vi "AddNewTSMProperty.vi"(9 "Target Class":path=path "GlobalTestData.lvclass", 10 "Property Scope":enum16{"Global", "PerSite"}(ring), 11 "Property Name":string) -> (0 "error out":errorcluster)   [LabVIEW 2019]
doc: "This VI will add a new Global (default) or Per-Site TSM-based property to the target class (default: GlobalTestData.lvclass). \nThis VI must be placed relative to the target class (same directory, or at a higher level).\nThis VI should not be added to, or claimed by, the target class (this is not the intended use case, you will get a lock-out error)."
uses:
  <vilib>/regexp/Match Regular Expression.xnode
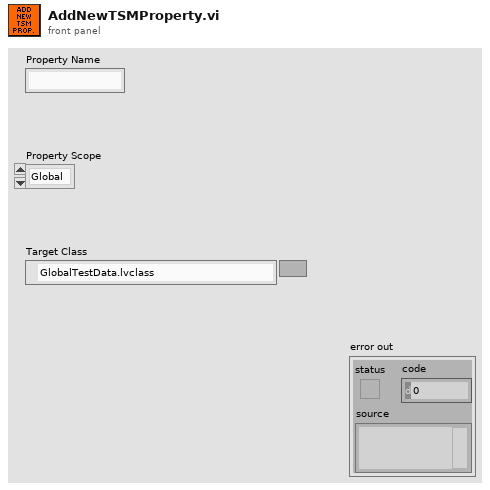
[diagram p1: front panel]
types:
  T1 = typedef "LIBUIP_item_type.ctl" = enum16{"None", "ParentLib", "Property Def Item", "VI", "Non-VI", "Folder", "Library", "Menu", "XI Ability VI", "XI Method VI", "XI Property VI", "Property Folder", "Class Private Data"}
  T2 = enum16{"Invalid Wire Rule", "Required", "Recommended", "Optional", "Dynamic Dispatch"}[]
  T3 = enum16{"Invalid Wire Rule", "Required", "Recommended", "Optional", "Dynamic Dispatch"}
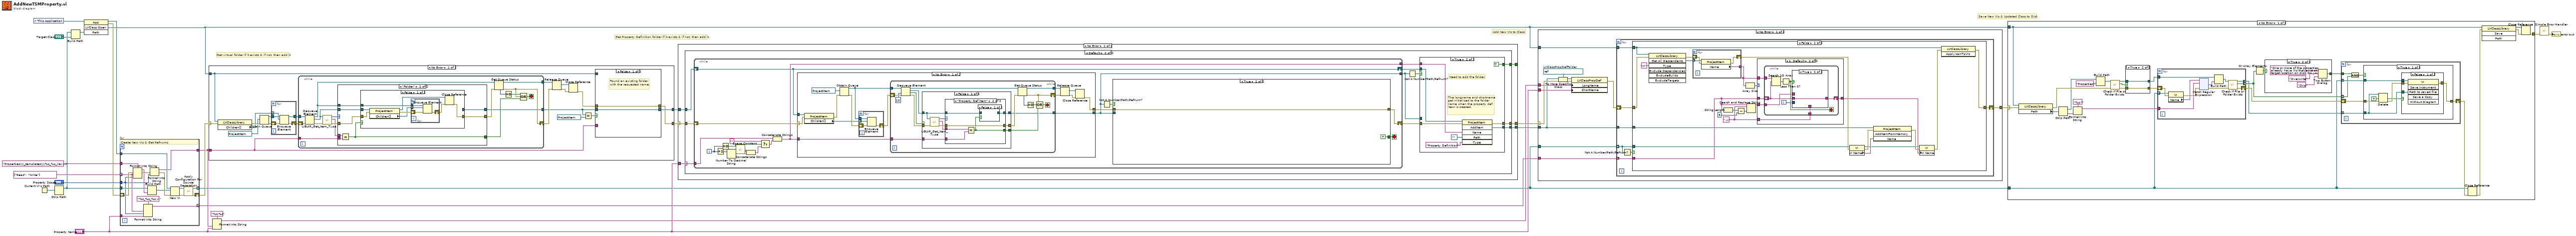
[diagram p0: block diagram]
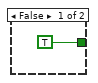
[diagram p2: hidden frame]
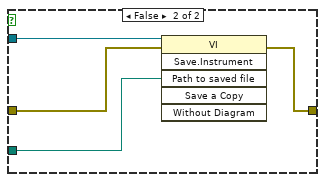
[diagram p4: hidden frame]
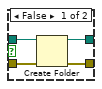
[diagram p5: hidden frame]
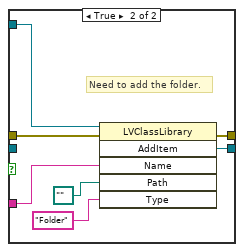
[diagram p7: hidden frame]
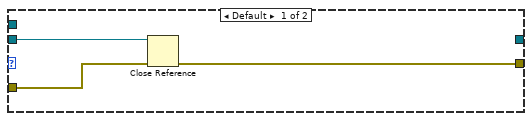
[diagram p8: hidden frame]
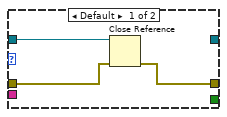
[diagram p12: hidden frame]
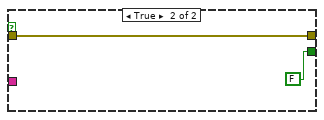
[diagram p14: hidden frame]
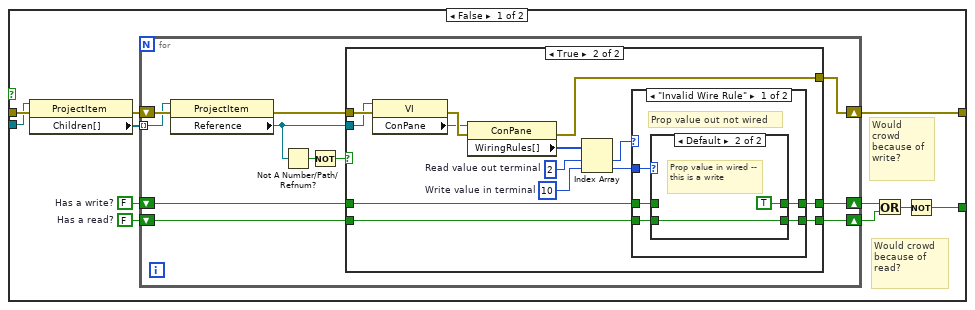
[diagram p16: hidden frame]
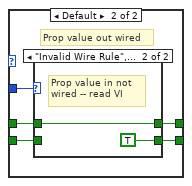
[diagram p19: hidden frame]
diagram:
  # "Add New VIs to Class"
  # "Save New VIs & Updated Class to Disk"
  # "Get Property Definition folder if it exists & if not, then add it"
  # "Get virtual folder if it exists & if not, then add it"
  n1 = control-ref of="This Application"() -> (w25:refnum<vi>)
  n2 = Current VI's Path() -> (path=w24:path)
  n3 = Strip Path(path=w24) -> (stripped path=w1:path)  [unwired: 1 out]
  n4 = Build Path(base path=w1, name or relative path="Target Class") -> (appended path=w3:path)
  n5 = invoke on="Invoke Node" class="App" method="LVClass.Open"(reference=w25, "Path"=w3) -> (reference out=w13:refnum<vi>, error out=w10:errorcluster, "LVClass.Open"=w16:refnum<vi>)  [unwired: 2 in, 1 out]
  n6 = for {
    tunnel: w1 -> [w42]
    tunnel: "Properties\\\\_templates\\\\%s_%s_Var.vit" -> [w41]
    tunnel: string[] ["Read", "Write"] -> [w31] mode=indexing
    tunnel: "Property Scope" -> [w30]
    tunnel: "Property Name" -> [w29]
    tunnel: w13 -> [w40]
    tunnel: [w39] -> w4 mode=indexing
    tunnel: [w35] -> w8
    shift-right: [w34] -> w15
    shift-left: w10 -> [w43]
    tunnel: [w27] -> w5 mode=indexing
    # "Create New VIs & Get Refnums"
    n7 = Format Into String(format string=w41, error in=w43, w31, w30) -> (resulting string=w28:string, error out=w38:errorcluster)  [unwired: 1 in]
    n8 = Format Into String(format string="%s_%s_%s.vi", w31, w30, w29) -> (resulting string=w27:string)  [unwired: 2 in, 1 out]
    n9 = Build Path(base path=w42, name or relative path=w28) -> (appended path=w33:path)
    n10 = Format Into String(error in=w38, w30) -> (resulting string=w35:string, error out=w37:errorcluster)  [unwired: 2 in]
    n11 = New VI(8:w37, 10:w33, 11:w40) -> (0:w26:errorcluster, 3:w36:refnum<vi>)  [unwired: 4 in]
    n12 = call <vilib>:"Apply Configuration For Source Separation.vi"("error in (no error)"=w26, "VI in"=w36) -> ("error out"=w34:errorcluster, "VI out"=w39:refnum<vi>)  [unwired: 8 in]
  }
  n13 = case shown="No Error" w15 {
    selector: w15 -> [w54 w120]
    tunnel: w8 -> [w45 _]
    tunnel: w16 -> [w44 _]
    tunnel: [w47 _] -> w23
    tunnel: [w46 w120] -> w22
    frame No Error {
      n14 = property class="LVClassLibrary"(reference=w44, error in=w54) -> (error out=w59:errorcluster, "Children[]"=w53:refnum<vi>[])  [unwired: 1 out]
      n15 = Obtain Queue(element data type=refnum<vi> refnum ("ProjectItem Refnum"), error in (no error)=w59) -> (queue out=w63:refnum<queue>, error out=w62:errorcluster)  [unwired: 2 in, 2 out]
      n16 = for {
        tunnel: w53 -> [w76] mode=indexing
        tunnel: w63 -> [w77]
        tunnel: [w73] -> w61
        shift-right: [w74] -> w60
        shift-left: w62 -> [w75]
        n17 = Enqueue Element(queue=w77, element=w76, error in (no error)=w75) -> (queue out=w73:refnum<queue>, error out=w74:errorcluster)  [unwired: 2 out]
      }
      n18 = while {
        tunnel: w61 -> [w92]
        shift-right: [w78] -> w55
        shift-left: w60 -> [w93]
        tunnel: [w79] -> w58
        tunnel: [w82] -> w49
        tunnel: w45 -> [w81]
        stop <- w88 stop-if-true
        n19 = Dequeue Element(queue=w92, error in (no error)=w93) -> (queue out=w83:refnum<queue>, element=w91:refnum<vi>, error out=w90:errorcluster)  [unwired: 2 out]
        n20 = call <resource>:"LIBUIP_Get_Item_Type.vi"("error in (no error)"=w90, "ProjectItem Refnum"=w91) -> ("error out"=w94:errorcluster, "Name"=w87:string, "Type"=w80:T1)  [unwired: 7 out]
        n21 = case shown="\"Folder\"" w80 {
          tunnel: [_ w104] -> w89
          tunnel: w87 -> [_ w105]
          tunnel: w91 -> [w97 w103]
          tunnel: w83 -> [_ w102]
          tunnel: w94 -> [w96 w101]
          tunnel: [w95 w100] -> w86
          tunnel: [_ w99] -> w82
          tunnel: w81 -> [_ w98]
          frame Default {
            n22 = Close Reference(reference=w97, error in (no error)=w96) -> (error out=w95:errorcluster)
          }
          frame "Folder" {
            n23 = Equal?(x=w105, y=w98) -> (x = y?=w104:bool)
            n24 = case shown="False" w104 {
              tunnel: w103 -> [w111 w118]
              tunnel: w102 -> [w110 _]
              tunnel: w101 -> [w113 w119]
              tunnel: [w107 w119] -> w100
              tunnel: [_ w118] -> w99
              frame False {
                n25 = property class="ProjectItem"(reference=w111, error in=w113) -> (reference out=w109:refnum<vi>, error out=w112:errorcluster, "Children[]"=w106:refnum<vi>[])
                n26 = for {
                  tunnel: w106 -> [w117] mode=indexing
                  tunnel: w110 -> [w116]
                  shift-right: [w114] -> w108
                  shift-left: w112 -> [w115]
                  n27 = Enqueue Element(queue=w116, element=w117, error in (no error)=w115) -> (error out=w114:errorcluster)  [unwired: 3 out]
                }
                n28 = Close Reference(reference=w109, error in (no error)=w108) -> (error out=w107:errorcluster)
              }
              frame True {
              }
            }
          }
        }
        n29 = Get Queue Status(queue=w83, error in (no error)=w86) -> (queue out=w79:refnum<queue>, error out=w78:errorcluster, # elements in queue=w85:i32)  [unwired: 6 out]
        n30 = Equal To 0?(x=w85) -> (x = 0?=w84:bool)
        n31 = Compound Arithmetic op=OR(w84, w78, w89) -> (w88:bool)
      }
      n32 = Release Queue(queue=w58, error in (no error)=w55) -> (remaining elements=w57:refnum<vi>[], error out=w56:errorcluster)  [unwired: 2 out]
      n33 = Close Reference(reference=w57, error in (no error)=w56) -> (error out=w48:errorcluster)
      n34 = Equal?(x=w49, y=refnum<vi> refnum ("ProjectItem Refnum")) -> (x = y?=w51:bool)
      n35 = case shown="False" w51 {
        tunnel: w49 -> [w65 _]
        tunnel: [w65 w66] -> w47
        tunnel: w44 -> [_ w72]
        tunnel: w45 -> [_ w71]
        tunnel: w48 -> [w64 w69]
        tunnel: [w64 w68] -> w46
        frame False {
          # "Found an existing folder with the requested name."
        }
        frame True {
          # "Need to add the folder."
          n36 = invoke class="LVClassLibrary" method="AddItem"(reference=w72, error in=w69, "Name"=w71, "Path"=path "", "Type"="Folder") -> (error out=w68:errorcluster, "AddItem"=w66:refnum<vi>)  [unwired: 1 in, 4 out]
        }
      }
    }
    frame Error {
    }
  }
  n37 = Format Into String(format string="%s:%s", w8, "Property Name") -> (resulting string=w6:string)  [unwired: 2 in, 1 out]
  n38 = case shown="No Error" w22 {
    selector: w22 -> [w123 w283]
    tunnel: [w122 w283] -> w19
    tunnel: w23 -> [w124 _]
    tunnel: "Property Name" -> [w126 _]
    tunnel: [w125 _] -> w17
    tunnel: [w121 _] -> _
    frame No Error {
      n39 = case shown="Default" w126 {
        selector: w126 -> [_ w132]
        tunnel: [w128 w139] -> w125
        tunnel: w124 -> [w128 w134]
        tunnel: w123 -> [w127 w133]
        tunnel: [w127 w137] -> w122
        tunnel: [_ w135] -> w121
        frame "" {
          # "If folder string is empty, just add at the top level (so the folder is the library itself)."
        }
        frame Default {
          n40 = while {
            tunnel: w132 -> [w154]
            shift-right: [w152] -> w138
            shift-left: w133 -> [w149]
            shift-right: [w147] -> w136
            shift-left: w134 -> [w147]
            tunnel: [w148] -> w129
            tunnel: [w150] -> w131
            i -> [w153]
            stop <- w155 stop-if-true
            n41 = Increment(x=w153) -> (x+1=w143:i32)
            n42 = Equal To 0?(x=w153) -> (x = 0?=w145:bool)
            n43 = Number To Decimal String(number=w143) -> (decimal integer string=w142:string)  [unwired: 1 in]
            n44 = call <vilib>:"Space Constant.vi"() -> ("String"=w141:string)
            n45 = Concatenate Strings(w141, w142) -> (w140:string)
            n46 = Select(t="" ("Proposed Property Folder Name"), s=w145, f=w140) -> (s? t:f=w144:string)
            n47 = Concatenate Strings(w154, w144) -> (w150:string)
            n48 = case shown="No Error" w149 {
              selector: w149 -> [w159 w213]
              tunnel: [w161 w213] -> w156
              tunnel: w147 -> [w170 _]
              tunnel: [w160 _] -> w148
              tunnel: w150 -> [w157 _]
              frame No Error {
                n49 = property class="ProjectItem"(reference=w170, error in=w159) -> (error out=w166:errorcluster, "Children[]"=w169:refnum<vi>[])  [unwired: 1 out]
                n50 = Obtain Queue(element data type=refnum<vi> refnum ("ProjectItem Refnum"), error in (no error)=w166) -> (queue out=w158:refnum<queue>, error out=w171:errorcluster)  [unwired: 2 in, 2 out]
                n51 = for {
                  tunnel: w169 -> [w211] mode=indexing
                  tunnel: w158 -> [w212]
                  shift-right: [w209] -> w167
                  shift-left: w171 -> [w210]
                  n52 = Enqueue Element(queue=w212, element=w211, error in (no error)=w210) -> (error out=w209:errorcluster)  [unwired: 3 out]
                }
                n53 = while {
                  shift-right: [w173] -> w162
                  shift-left: w167 -> [w187]
                  tunnel: [w175] -> w165
                  tunnel: [w179] -> w160
                  tunnel: w158 -> [w178]
                  tunnel: w157 -> [w172]
                  stop <- w183 stop-if-true
                  n54 = Dequeue Element(queue=w178, timeout in ms (-1)=10, error in (no error)=w187) -> (queue out=w180:refnum<queue>, element=w186:refnum<vi>, timed out?=w176:bool, error out=w185:errorcluster)
                  n55 = case shown="False" w176 {
                    tunnel: w186 -> [w196 _]
                    tunnel: w185 -> [w195 w207]
                    tunnel: [w191 FALSE] -> w184
                    tunnel: [w193 w207] -> w182
                    tunnel: [w192 _] -> w179
                    tunnel: w172 -> [w188 _]
                    frame False {
                      n56 = call <resource>:"LIBUIP_Get_Item_Type.vi"("error in (no error)"=w195, "ProjectItem Refnum"=w196) -> ("error out"=w194:errorcluster, "Name"=w189:string, "Type"=w190:T1)  [unwired: 7 out]
                      n57 = case shown="\"Property Def Item\"" w190 {
                        tunnel: w189 -> [_ w205]
                        tunnel: w196 -> [w199 w204]
                        tunnel: w194 -> [w198 w202]
                        tunnel: [w197 w202] -> w193
                        tunnel: [_ w203] -> w192
                        tunnel: [_ w200] -> w191
                        tunnel: w188 -> [_ w201]
                        frame Default {
                          n58 = Close Reference(reference=w199, error in (no error)=w198) -> (error out=w197:errorcluster)
                        }
                        frame "Property Def Item" {
                          n59 = Equal?(x=w205, y=w201) -> (x = y?=w200:bool)
                          n60 = case shown="False" w200 {
                            tunnel: w204 -> [_ w206]
                            tunnel: [_ w206] -> w203
                            frame False {
                            }
                            frame True {
                            }
                          }
                        }
                      }
                    }
                    frame True {
                    }
                  }
                  n61 = Get Queue Status(queue=w180, error in (no error)=w182) -> (queue out=w175:refnum<queue>, error out=w173:errorcluster, # elements in queue=w181:i32)  [unwired: 6 out]
                  n62 = Equal To 0?(x=w181) -> (x = 0?=w174:bool)
                  n63 = Compound Arithmetic op=OR(w173, w174, w184) -> (w183:bool)
                }
                n64 = Release Queue(queue=w165, error in (no error)=w162) -> (remaining elements=w164:refnum<vi>[], error out=w163:errorcluster)  [unwired: 2 out]
                n65 = Close Reference(reference=w164, error in (no error)=w163) -> (error out=w161:errorcluster)
              }
              frame Error {
              }
            }
            n66 = Not A Number/Path/Refnum?(number/path/refnum=w148) -> (NaN/Path/Refnum?=w151:bool)
            n67 = case shown="True" w151 {
              tunnel: [w224 TRUE] -> w155
              tunnel: w156 -> [w219 w272]
              tunnel: [w217 w272] -> w152
              tunnel: w148 -> [w216 _]
              frame False {
                w222 = FALSE  # Has a read?
                w221 = FALSE  # Has a write?
                # "Would crowd because of read?"
                # "Would crowd because of write?"
                n68 = property class="ProjectItem"(reference=w216, error in=w219) -> (error out=w223:errorcluster, "Children[]"=w220:refnum<vi>[])  [unwired: 1 out]
                n69 = for {
                  tunnel: w220 -> [w227] mode=indexing
                  shift-right: [w233] -> w215
                  shift-left: w221 -> [w232]
                  shift-right: [w231] -> w214
                  shift-left: w222 -> [w230]
                  shift-right: [w225] -> w217
                  shift-left: w223 -> [w229]
                  n70 = property class="ProjectItem"(reference=w227, error in=w229) -> (error out=w228:errorcluster, "Reference"=w226:refnum<vi>)  [unwired: 1 out]
                  n71 = Not A Number/Path/Refnum?(number/path/refnum=w226) -> (NaN/Path/Refnum?=w235:bool)
                  n72 = Not(x=w235) -> (.not. x?=w234:bool)
                  n73 = case shown="True" w234 {
                    tunnel: w226 -> [_ w239]
                    tunnel: [w238 w245] -> w233
                    tunnel: w232 -> [w238 w244]
                    tunnel: [w237 w243] -> w231
                    tunnel: w230 -> [w237 w242]
                    tunnel: w228 -> [w236 w241]
                    tunnel: [w236 w240] -> w225
                    frame False {
                    }
                    frame True {
                      w248 = 10  # Write value in terminal
                      w249 = 2  # Read value out terminal
                      n74 = property class="VI"(reference=w239, error in=w241) -> (error out=w252:errorcluster, "ConPane"=w251:refnum<vi>)  [unwired: 1 out]
                      n75 = property class="ConPane"(reference=w251, error in=w252) -> (error out=w240:errorcluster, "WiringRules[]"=w250:T2)  [unwired: 1 out]
                      n76 = Index Array(array=w250, index #1=w249, index #2=w248) -> (element #1=w247:T3, element #2=w246:T3)
                      n77 = case shown="\"Invalid Wire Rule\"" w247 {
                        tunnel: w246 -> [w257 w266]
                        tunnel: [w256 w262] -> w245
                        tunnel: w244 -> [w255 w263]
                        tunnel: [w253 w265] -> w243
                        tunnel: w242 -> [w254 w264]
                        frame "Invalid Wire Rule" {
                          # "Prop value out not wired"
                          n78 = case shown="Default" w257 {
                            tunnel: [w259 TRUE] -> w256
                            tunnel: w255 -> [w259 _]
                            tunnel: w254 -> [w258 w260]
                            tunnel: [w258 w260] -> w253
                            frame "Invalid Wire Rule" {
                              # "Neither wired...bad vi"
                            }
                            frame Default {
                              # "Prop value in wired -- this is a write"
                            }
                          }
                        }
                        frame Default {
                          # "Prop value out wired"
                          n79 = case shown="\"Invalid Wire Rule\", \"Optional\"" w266 {
                            tunnel: [w267 TRUE] -> w265
                            tunnel: w264 -> [w267 _]
                            tunnel: w263 -> [w268 w269]
                            tunnel: [w268 w269] -> w262
                            frame Default {
                              # "Both wired...bad"
                            }
                            frame "Invalid Wire Rule", "Optional" {
                              # "Prop value in not wired -- read VI"
                            }
                          }
                        }
                      }
                    }
                  }
                }
                n80 = Or(x=w215, y=w214) -> (x .or. y?=w218:bool)
                n81 = Not(x=w218) -> (.not. x?=w224:bool)
              }
              frame True {
              }
            }
          }
          n82 = Not A Number/Path/Refnum?(number/path/refnum=w129) -> (NaN/Path/Refnum?=w130:bool)
          n83 = case shown="True" w130 {
            tunnel: w136 -> [_ w279]
            tunnel: [w273 w275] -> w139
            tunnel: w131 -> [_ w277]
            tunnel: w138 -> [w274 w281]
            tunnel: [w274 w276] -> w137
            tunnel: w129 -> [w273 _]
            tunnel: [_ TRUE] -> w135
            frame False {
              # "Found an existing folder with the requested name."
            }
            frame True {
              # "The longname and shortname get initialized to the folder name when the property def item is created."
              # "Need to add the folder."
              n84 = invoke class="ProjectItem" method="AddItem"(reference=w279, error in=w281, "Name"=w277, "Path"=path "", "Type"="Property Definition") -> (error out=w276:errorcluster, "AddItem"=w275:refnum<vi>)  [unwired: 1 in, 4 out]
            }
          }
        }
      }
    }
    frame Error {
    }
  }
  n85 = case shown="No Error" w19 {
    selector: w19 -> [w291 w353]
    tunnel: [w284 w353] -> w18
    tunnel: w17 -> [w286 _]
    tunnel: w16 -> [w285 _]
    tunnel: w6 -> [w290 _]
    tunnel: "Property Name" -> [w289 _]
    tunnel: w4 -> [w288 _]
    tunnel: w5 -> [w287 _]
    frame No Error {
      w292 = refnum<vi> refnum  # LVClassPropDefFolder
      n86 = To More Specific Class(target class=w292, reference=w286, error in=w291) -> (specific class reference=w293:refnum<vi>, error out=w294:errorcluster)
      n87 = property class="LVClassPropDef"(reference=w293, error in=w294, "LongName"=w290, "ShortName"=w289) -> (error out=w295:errorcluster)  [unwired: 1 out]
      n88 = for {
        tunnel: w288 -> [w297] mode=indexing
        shift-right: [w300] -> w284
        shift-left: w295 -> [w301]
        tunnel: w287 -> [w298] mode=indexing
        tunnel: w286 -> [w299]
        tunnel: w285 -> [w296]
        n89 = Not A Number/Path/Refnum?(number/path/refnum=w297) -> (NaN/Path/Refnum?=w302:bool)
        n90 = case shown="False" w302 {
          tunnel: w301 -> [w305 w352]
          tunnel: [w320 w352] -> w300
          tunnel: w299 -> [w318 _]
          tunnel: w298 -> [w304 _]
          tunnel: w297 -> [w319 _]
          tunnel: w296 -> [w306 _]
          frame False {
            w308 = ".vi" ("search string")
            n91 = invoke class="LVClassLibrary" method="Get All Descendents"(reference=w306, error in=w305, "Type"="VI") -> (error out=w315:errorcluster, "All Descendents"=w316:refnum<vi>[])  [unwired: 4 in, 5 out]
            n92 = for {
              tunnel: w316 -> [w351] mode=indexing
              shift-right: [w349] -> w307
              shift-left: w315 -> [w350]
              tunnel: [w348] -> w314 mode=indexing
              n93 = property class="ProjectItem"(reference=w351, error in=w350) -> (error out=w349:errorcluster, "Name"=w348:string)  [unwired: 1 out]
            }
            n94 = String Length(string=w304) -> (length=w312:i32)
            n95 = Subtract(x=w312, y=3) -> (x-y=w311:i32)
            n96 = Array Size(array=w314) -> (size(s)=w313:i32)
            n97 = Search and Replace String(input string=w304, search string=w308, offset=w311) -> (result string=w309:string)  [unwired: 1 in, 7 out]
            n98 = case shown="1, Default" w313 {
              tunnel: w314 -> [_ w331]
              tunnel: w304 -> [w326 w330]
              tunnel: [w326 w329] -> w303
              tunnel: w309 -> [_ w328]
              tunnel: w308 -> [_ w327]
              frame 0 {
              }
              frame 1, Default {
                n99 = while {
                  tunnel: w331 -> [w339]
                  shift-right: [w337] -> w329
                  shift-left: w330 -> [w336]
                  tunnel: w328 -> [w334]
                  tunnel: w327 -> [w332]
                  i -> [w333]
                  stop <- w335 stop-if-true
                  n100 = Search 1D Array(1D array=w339, element=w336) -> (index of element=w338:i32)  [unwired: 1 out]
                  n101 = Less Than 0?(x=w338) -> (x < 0?=w335:bool)
                  n102 = case shown="True" w335 {
                    tunnel: [w344 w347] -> w337
                    tunnel: w336 -> [_ w347]
                    tunnel: w334 -> [w345 _]
                    tunnel: w333 -> [w346 _]
                    tunnel: w332 -> [w341 _]
                    frame False {
                      n103 = Add(x=w346, y=2) -> (x+y=w343:i32)
                      n104 = Format Into String(format string="%s %d%s", w345, w343, w341) -> (resulting string=w344:string)  [unwired: 2 in, 1 out]
                    }
                    frame True {
                    }
                  }
                }
              }
            }
            n105 = property on="Property Node" class="VI"(reference=w319, error in=w307) -> (reference out=w321:refnum<vi>, error out=w324:errorcluster, "VI Name"=w323:string)
            n106 = invoke on="Invoke Node" class="ProjectItem" method="AddItemFromMemory"(reference=w318, error in=w324, "Name"=w323) -> (error out=w322:errorcluster)  [unwired: 1 in, 3 out]
            n107 = property on="Property Node" class="VI"(reference=w321, error in=w322, "VI Name"=w303) -> (error out=w325:errorcluster)  [unwired: 1 out]
            n108 = invoke class="LVClassLibrary" method="ApplyIconToVIs"(reference=w306, error in=w325) -> (error out=w320:errorcluster)  [unwired: 1 in, 2 out]
          }
          frame True {
          }
        }
      }
    }
    frame Error {
    }
  }
  n109 = case shown="No Error" w18 {
    selector: w18 -> [w377 w540]
    tunnel: w4 -> [w359 _]
    tunnel: w16 -> [w376 _]
    tunnel: [w363 w540] -> w21
    frame No Error {
      n110 = property class="LVClassLibrary"(reference=w376, error in=w377) -> (error out=w372:errorcluster, "Path"=w371:path)  [unwired: 1 out]
      n111 = Strip Path(path=w371) -> (stripped path=w362:path, name=w369:string)
      n112 = Format Into String(format string="%s:*", w369) -> (resulting string=w370:string)  [unwired: 2 in, 1 out]
      n113 = Build Path(base path=w362, name or relative path="Properties") -> (appended path=w357:path)
      n114 = call <vilib>:"Check if File or Folder Exists.vi"("error in (no error)"=w372, "path"=w357) -> ("error out"=w356:errorcluster, "file or folder exists?"=w354:bool, "dup path"=w355:path)  [unwired: 7 in]
      n115 = case shown="True" w354 {
        tunnel: w356 -> [w537 w539]
        tunnel: [w536 w539] -> w374
        tunnel: w355 -> [w535 w538]
        tunnel: [w534 w538] -> w373
        frame False {
          n116 = Create Folder(path (use dialog)=w535, error in=w537) -> (created path=w534:path, error out=w536:errorcluster)  [unwired: 1 in, 1 out]
        }
        frame True {
        }
      }
      n117 = for {
        tunnel: w359 -> [w393] mode=indexing
        shift-right: [w387] -> w367
        shift-left: w374 -> [w395]
        tunnel: w373 -> [w394]
        tunnel: w370 -> [w391]
        tunnel: [w388] -> w361 mode=indexing
        tunnel: [w386] -> w364 mode=indexing
        n118 = property class="VI"(reference=w393, error in=w395) -> (error out=w396:errorcluster, "Name"=w385:string)  [unwired: 1 out]
        n119 = xnode "Match Regular Expression"("input string"=w385, "regular expression"=w391, "error in"=w396) -> ("after match"=w392:string, "error out"=w390:errorcluster)  [unwired: 3 in, 3 out]
        n120 = Build Path(base path=w394, name or relative path=w392) -> (appended path=w389:path)
        n121 = call <vilib>:"Check if File or Folder Exists.vi"("error in (no error)"=w390, "path"=w389) -> ("error out"=w387:errorcluster, "file or folder exists?"=w386:bool, "dup path"=w388:path)  [unwired: 7 in]
      }
      n122 = Or Array Elements(Boolean array=w364) -> (logical OR=w365:bool)
      n123 = case shown="True" w365 {
        tunnel: [TRUE ("T button?") w384] -> w360
        frame False {
        }
        frame True {
          n124 = Two Button Dialog(message="One or more of the properties already have VIs that exist at the target location on disk. Do you want to override those VIs or skip them?", 1:"Skip" ("T button name (\"OK\")"), 2:"Overwrite" ("T button name (\"OK\")")) -> (T button?=w384:bool)
        }
      }
      n125 = for {
        shift-right: [w517] -> w366
        shift-left: w367 -> [w514]
        tunnel: w359 -> [w516] mode=indexing
        tunnel: w361 -> [w515] mode=indexing
        tunnel: w364 -> [w513] mode=indexing
        tunnel: w360 -> [w512]
        n126 = And(x=w512, y=w513) -> (x .and. y?=w511:bool)
        n127 = case shown="True" w511 {
          tunnel: [w524 w533] -> w517
          tunnel: w516 -> [w523 w532]
          tunnel: w515 -> [w520 w531]
          tunnel: w514 -> [w522 w530]
          frame True {
            n128 = Delete(path (use dialog)=w520, confirm (F)=TRUE, error in=w522) -> (cancelled=w518:bool, error out=w521:errorcluster)  [unwired: 2 in, 1 out]
            n129 = case shown="False" w518 {
              tunnel: [w528 w529] -> w524
              tunnel: w523 -> [w527 _]
              tunnel: w521 -> [w526 w529]
              tunnel: w520 -> [w525 _]
              frame False {
                n130 = invoke class="VI" method="Save.Instrument"(reference=w527, error in=w526, "Path to saved file"=w525) -> (error out=w528:errorcluster)  [unwired: 3 in, 5 out]
              }
              frame True {
              }
            }
          }
          frame False {
            n131 = invoke class="VI" method="Save.Instrument"(reference=w532, error in=w530, "Path to saved file"=w531) -> (error out=w533:errorcluster)  [unwired: 3 in, 5 out]
          }
        }
      }
      n132 = Close Reference(reference=w359, error in (no error)=w366) -> (error out=w375:errorcluster)
      n133 = invoke class="LVClassLibrary" method="Save"(reference=w376, error in=w375) -> (reference out=w378:refnum<vi>, error out=w379:errorcluster)  [unwired: 2 in, 2 out]
      n134 = Close Reference(reference=w378, error in (no error)=w379) -> (error out=w363:errorcluster)
    }
    frame Error {
    }
  }
  n135 = call <vilib>:"Simple Error Handler.vi"("error in (no error)"=w21) -> ("error out"=→"error out":errorcluster)  [unwired: 4 in, 4 out]
